vi "Begin.vi"(8 "error in":errorcluster) -> (0 "error out":errorcluster)   [LabVIEW 2017]
doc: "Called before other user functions, this VI is expected to open initial I/O refnums, load in file data, and do all program initialization. Notice that the <B>error out</B> terminal is simply used for data flow. Wiring it to other structures or subVIs ensures that this VI runs first."
uses:
  <vilib>/Rock Robotics/WPI/DriverStation/WPI_DriverStationRobotMode2.ctl
  TypeDef/CLUSTER_Arm_Device_IDs.ctl
  TypeDef/CLUSTER_Talon_Setup.ctl
  _SHARE ALL/RoboRio Share All/SRX Share All/TypeDefs SRX/Cluster_SRX_OPEN Data.ctl
  _SHARE ALL/RoboRio Share All/SRX Share All/TypeDefs SRX/Cluster_SRX_Current Config.ctl
  _SHARE ALL/RoboRio Share All/SRX Share All/TypeDefs SRX/Cluster_SRX_Sensor Config.ctl
  System Drivers/Phoenix-LabVIEW/Motor Controller/Controls/CTRE_Phoenix_MotorControl_FeedbackDevice.ctl
  _SHARE ALL/RoboRio Share All/SRX Share All/TypeDefs SRX/Cluster_SRX_Config Hard Limits.ctl
  System Drivers/Phoenix-LabVIEW/Motor Controller/Controls/CTRE_Phoenix_MotorControl_LimitSwitchNormal.ctl
  _SHARE ALL/RoboRio Share All/SRX Share All/TypeDefs SRX/Cluster_SRX_Motion Magic Config Data.ctl
  _SHARE ALL/RoboRio Share All/SRX Share All/TypeDefs SRX/Cluster_SRX_PIDF.ctl
  _SHARE ALL/RoboRio Share All/SRX Share All/TypeDefs SRX/Cluster_SRX_Config Soft Limits.ctl
  _SHARE ALL/RoboRio Share All/SRX Share All/TypeDefs SRX/Cluster_SRX_Config Voltage Output.ctl
  System Drivers/Phoenix-LabVIEW/Motor Controller/Controls/CTRE_Phoenix_MotorControl_NeutralMode.ctl
  _SHARE ALL/RoboRio Share All/SRX Share All/TypeDefs SRX/Cluster_SRX_Forward and Reverse.ctl
  TypeDef/CLUSTER_Claw_Setup.ctl
  TypeDef/CLUSTER_PWM Motor Setup.ctl
  <vilib>/Rock Robotics/SystemInterfaces/DIO/FPGA_DIOPWMChannel.ctl
  TypeDef/CLUSTER_Solonoid_Setup.ctl
  <vilib>/Rock Robotics/WPI/Solenoid/WPI_SolenoidChannel.ctl
  <vilib>/Rock Robotics/SystemInterfaces/DIO/FPGA_DIOChannel.ctl
  Robot Global Data.vi
  _SHARE ALL/Global Share All/Global_STOP.vi
  Globals/Global_Device_IDs.vi
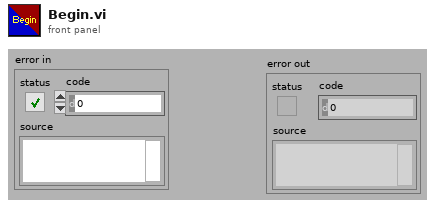
[diagram p1: front panel]
types:
  T1 = typedef "WPI_DriverStationRobotMode2.ctl" = enum16{"Autonomous Disabled", "Autonomous Enabled", "Teleop Disabled", "Teleop Enabled", "Disconnected", "Finish", "Test Disabled", "Test Enabled", "Emergency Stopped"}
  T2 = typedef "Cluster_SRX_Forward and Reverse.ctl" = cluster{"Forward":dbl, "Reverse":dbl}
  T3 = typedef "CTRE_Phoenix_MotorControl_NeutralMode.ctl" = enum8{"EEPROMSetting", "Override to Coast", "Override to Brake"}
  T4 = typedef "Cluster_SRX_Config Voltage Output.ctl" = cluster{"Invert?":bool, "Neutral Mode":T3, "Deadband (-1to1)":dbl, "Ramp Time Off to Full (S)":dbl, "Peak  (-1to1)":T2, "Nominal  (-1to1)":T2}
  T5 = typedef "Cluster_SRX_Config Soft Limits.ctl" = cluster{"Max":i32, "Min":i32, "Max Enable":bool, "Min Enable":bool}
  T6 = typedef "Cluster_SRX_PIDF.ctl" = cluster{"P":dbl, "I":dbl, "D":dbl, "F":dbl, "I Zone":dbl}
  T7 = typedef "Cluster_SRX_Sensor Config.ctl" = cluster{"Feedback Device":T8, "PhaseSensor":bool}
  T8 = typedef "CTRE_Phoenix_MotorControl_FeedbackDevice.ctl" = i8
  T9 = typedef "Cluster_SRX_OPEN Data.ctl" = cluster{"SRX ID":u8, "Invert Output":bool}
  T10 = typedef "CLUSTER_Talon_Setup.ctl" = cluster{"Open Data":T9, "Current Config Data":T11, "Sensor Config":T7, "Hard Limits":T12, "Motion Magic Config Data":T14, "PIDF":T6, "Maximum Integral Accumulator Value":dbl, "AllowableClosedLoop":i32, "Limits":T5, "Output Config":T4}
  T11 = typedef "Cluster_SRX_Current Config.ctl" = cluster{"Enable Current Limit?":bool, "Peak Current (Amps)":i32, "Peak Current Maximum Duration (ms)":i32, "Continuous Current Limit (Amps)":i32}
  T12 = typedef "Cluster_SRX_Config Hard Limits.ctl" = cluster{"Fwd Enable":bool, "Rev Enable":bool, "Fwd NO-NC":T13, "Rev NO-NC":T13}
  T13 = typedef "CTRE_Phoenix_MotorControl_LimitSwitchNormal.ctl" = enum16{"Normally Open", "Normally Closed", "Disabled"}
  T14 = typedef "Cluster_SRX_Motion Magic Config Data.ctl" = cluster{"Cruise Velocity":i32, "Acceleration":i32}
  T15 = typedef "CLUSTER_Arm_Device_IDs.ctl" = cluster{"Master":T10, "Slave":T10}
  T16 = typedef "FPGA_DIOChannel.ctl" = enum8{"DIO 0", "DIO 1", "DIO 2", "DIO 3", "DIO 4", "DIO 5", "DIO 6", "DIO 7", "DIO 8", "DIO 9", "DIO MXP 0", "DIO MXP 1", "DIO MXP 2", "DIO MXP 3", "DIO MXP 4", "DIO MXP 5", "DIO MXP 6", "DIO MXP 7", "DIO MXP 8", "DIO MXP 9", "DIO MXP 10", "DIO MXP 11", "DIO MXP 12", "DIO MXP 13", "DIO MXP 14", "DIO MXP 15", "SPI Port CS1", "SPI Port CS2", "SPI Port CS3", "SPI Port MISO", "SPI Port MOSI", "Invalid"}
  T17 = typedef "WPI_SolenoidChannel.ctl" = enum8{"Solenoid 0", "Solenoid 1", "Solenoid 2", "Solenoid 3", "Solenoid 4", "Solenoid 5", "Solenoid 6", "Solenoid 7", "Invalid"}
  T18 = typedef "FPGA_DIOPWMChannel.ctl" = enum8{"PWM 0", "PWM 1", "PWM 2", "PWM 3", "PWM 4", "PWM 5", "PWM 6", "PWM 7", "PWM 8", "PWM 9", "PWM MXP 0", "PWM MXP 1", "PWM MXP 2", "PWM MXP 3", "PWM MXP 4", "PWM MXP 5", "PWM MXP 6", "PWM MXP 7", "PWM MXP 8", "PWM MXP 9", "Invalid"}
  T19 = typedef "CLUSTER_Claw_Setup.ctl" = cluster{"Left Motor Setup":T20, "Right Motor Setup":T20, "Left Motor PDP":i32, "Right Motor PDP":i32, "Solonoid Setup":T21, "Limit Switch DIO":T16}
  T20 = typedef "CLUSTER_PWM Motor Setup.ctl" = cluster{"Motor PWM":T18, "Invert Motor":bool}
  T21 = typedef "CLUSTER_Solonoid_Setup.ctl" = cluster{"Pneumatics Control Module (0)":u8, "Forward Solenoid Channel":T17, "Reverse Solenoid Channel":T17}
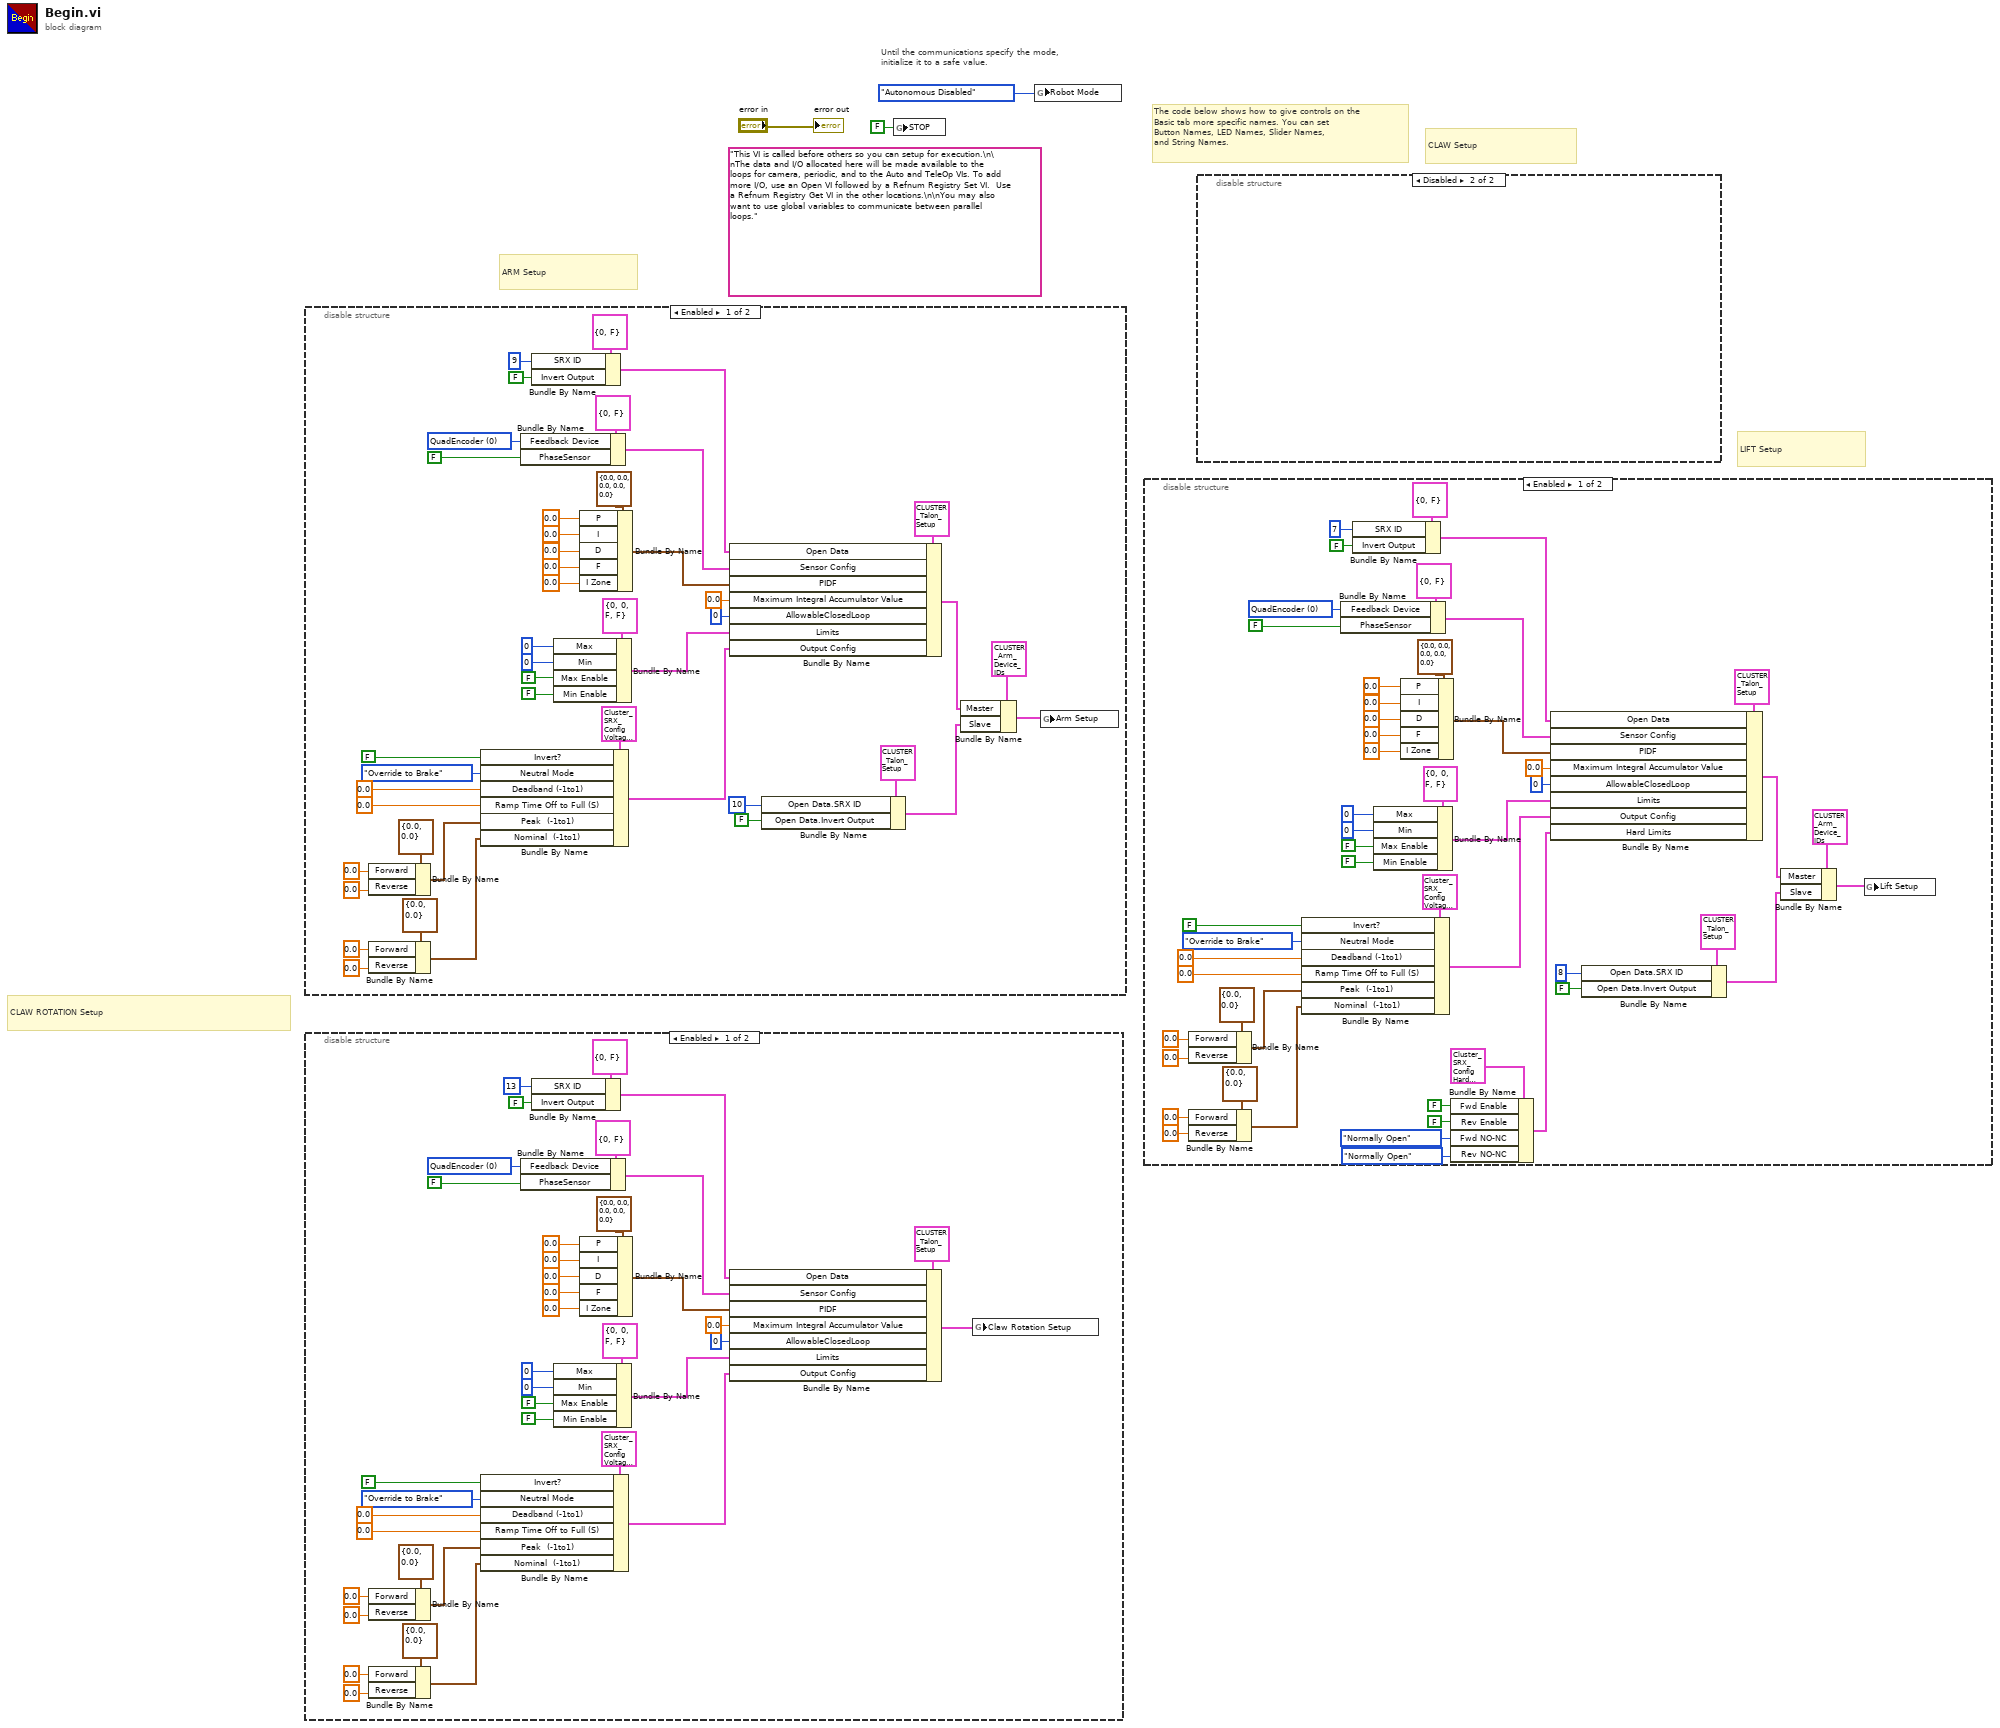
[diagram p0: block diagram]
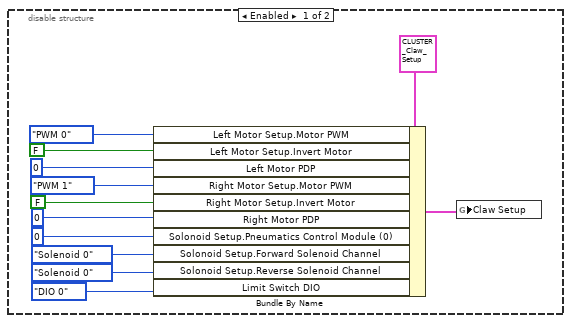
[diagram p4: hidden frame]
diagram:
  (unwired) "This VI is called before others so you can setup for execution.\n\nThe data and I/O allocated here will be made available to the loops for camera, periodic, and to the Auto and TeleOp VIs. To add more I/O, use an Open VI followed by a Refnum Registry Set VI.  Use a Refnum Registry Get VI in the other locations.\n\nYou may also want to use global variables to communicate between parallel loops."
  # "CLAW ROTATION Setup"
  # "LIFT Setup"
  # "CLAW Setup"
  # "ARM Setup"
  # "The code below shows how to give controls on the\nBasic tab more specific names. You can set\nButton Names, LED Names, Slider Names,\nand String Names."
  # "Until the communications specify the mode,\ninitialize it to a safe value."
  n1 = disable-structure shown="Enabled" {
    frame Enabled {
      w28 = T8 0 items=["None"=-1, "QuadEncoder"=0, "Analog"=2, "Tachometer"=4, "Pulse Width Encoded Position"=8, "Sensor Sum (S0 + S1)"=9, "Sensor Difference (D0 - D1)"=10, "Remote Source 0"=11, "Remote Source 1"=12, "Software Emulated"=15] ("Feedback Device")
      n2 = Bundle By Name(cluster=T2 {"Forward"=0.0, "Reverse"=0.0} ("Peak  (-1to1)"), "Forward"=0.0, "Reverse"=0.0) -> (w12:T2)
      n3 = Bundle By Name(cluster=T2 {"Forward"=0.0, "Reverse"=0.0} ("Nominal  (-1to1)"), "Forward"=0.0, "Reverse"=0.0) -> (w10:T2)
      n4 = Bundle By Name(cluster=T4 {"Invert?"=FALSE, "Neutral Mode"=enum."Override to Coast", "Deadband (-1to1)"=0.0, "Ramp Time Off to Full (S)"=0.0, "Peak  (-1to1)"={"Forward"=1.0, "Reverse"=-1.0}, "Nominal  (-1to1)"={"Forward"=0.0, "Reverse"=0.0}} ("Output Config"), "Invert?"=FALSE, "Neutral Mode"=CTRE_Phoenix_MotorControl_NeutralMode."Override to Brake", "Deadband (-1to1)"=0.0, "Ramp Time Off to Full (S)"=0.0, "Peak  (-1to1)"=w12, "Nominal  (-1to1)"=w10) -> (w31:T4)
      n5 = Bundle By Name(cluster=T7 {"Feedback Device"=0, "PhaseSensor"=FALSE} ("Sensor Config"), "Feedback Device"=w28, "PhaseSensor"=FALSE) -> (w39:T7)
      n6 = Bundle By Name(cluster=T9 {"SRX ID"=0, "Invert Output"=FALSE} ("Open Data"), "SRX ID"=u8 9, "Invert Output"=FALSE) -> (w41:T9)
      n7 = Bundle By Name(cluster=T5 {"Max"=0, "Min"=0, "Max Enable"=FALSE, "Min Enable"=FALSE} ("Limits"), "Max"=0, "Min"=0, "Max Enable"=FALSE, "Min Enable"=FALSE) -> (w33:T5)
      n8 = Bundle By Name(cluster=T6 {"P"=0.0, "I"=0.0, "D"=0.0, "F"=0.0, "I Zone"=0.0} ("PIDF"), "P"=0.0, "I"=0.0, "D"=0.0, "F"=0.0, "I Zone"=0.0) -> (w37:T6)
      n9 = Bundle By Name(cluster=T10 {"Open Data"={"SRX ID"=0, "Invert Output"=FALSE}, "Current Config Data"={"Enable Current Limit?"=FALSE, "Peak Current (Amps)"=0, "Peak Current Maximum Duration (ms)"=0, "Continuous Current Limit (Amps)"=0}, "Sensor Config"={"Feedback Device"=0, "PhaseSensor"=FALSE}, "Hard Limits"={"Fwd Enable"=FALSE, "Rev Enable"=FALSE, "Fwd NO-NC"=enum."Normally Open", "Rev NO-NC"=enum."Normally Open"}, "Motion Magic Config Data"={"Cruise Velocity"=0, "Acceleration"=0}, "PIDF"={"P"=0.0, "I"=0.0, "D"=0.0, "F"=0.0, "I Zone"=0.0}, "Maximum Integral Accumulator Value"=0.0, "AllowableClosedLoop"=0, "Limits"={"Max"=0, "Min"=0, "Max Enable"=FALSE, "Min Enable"=FALSE}, "Output Config"={"Invert?"=FALSE, "Neutral Mode"=enum."Override to Coast", "Deadband (-1to1)"=0.0, "Ramp Time Off to Full (S)"=0.0, "Peak  (-1to1)"={"Forward"=1.0, "Reverse"=-1.0}, "Nominal  (-1to1)"={"Forward"=0.0, "Reverse"=0.0}}} ("Master"), "Open Data"=w41, "Sensor Config"=w39, "PIDF"=w37, "Maximum Integral Accumulator Value"=0.0, "AllowableClosedLoop"=0, "Limits"=w33, "Output Config"=w31) -> (w45:T10)
      n10 = Bundle By Name(cluster=T10 {"Open Data"={"SRX ID"=0, "Invert Output"=FALSE}, "Current Config Data"={"Enable Current Limit?"=FALSE, "Peak Current (Amps)"=0, "Peak Current Maximum Duration (ms)"=0, "Continuous Current Limit (Amps)"=0}, "Sensor Config"={"Feedback Device"=0, "PhaseSensor"=FALSE}, "Hard Limits"={"Fwd Enable"=FALSE, "Rev Enable"=FALSE, "Fwd NO-NC"=enum."Normally Open", "Rev NO-NC"=enum."Normally Open"}, "Motion Magic Config Data"={"Cruise Velocity"=0, "Acceleration"=0}, "PIDF"={"P"=0.0, "I"=0.0, "D"=0.0, "F"=0.0, "I Zone"=0.0}, "Maximum Integral Accumulator Value"=0.0, "AllowableClosedLoop"=0, "Limits"={"Max"=0, "Min"=0, "Max Enable"=FALSE, "Min Enable"=FALSE}, "Output Config"={"Invert?"=FALSE, "Neutral Mode"=enum."Override to Coast", "Deadband (-1to1)"=0.0, "Ramp Time Off to Full (S)"=0.0, "Peak  (-1to1)"={"Forward"=1.0, "Reverse"=-1.0}, "Nominal  (-1to1)"={"Forward"=0.0, "Reverse"=0.0}}} ("Master"), "Open Data.SRX ID"=u8 10, "Open Data.Invert Output"=FALSE) -> (w44:T10)
      n11 = Bundle By Name(cluster=T15 {"Master"={"Open Data"={"SRX ID"=0, "Invert Output"=FALSE}, "Current Config Data"={"Enable Current Limit?"=FALSE, "Peak Current (Amps)"=0, "Peak Current Maximum Duration (ms)"=2, "Continuous Current Limit (Amps)"=0}, "Sensor Config"={"Feedback Device"=0, "PhaseSensor"=FALSE}, "Hard Limits"={"Fwd Enable"=FALSE, "Rev Enable"=FALSE, "Fwd NO-NC"=enum."Normally Open", "Rev NO-NC"=enum."Normally Open"}, "Motion Magic Config Data"={"Cruise Velocity"=0, "Acceleration"=0}, "PIDF"={"P"=0.0, "I"=0.0, "D"=0.0, "F"=0.0, "I Zone"=0.0}, "Maximum Integral Accumulator Value"=0.0, "AllowableClosedLoop"=0, "Limits"={"Max"=0, "Min"=0, "Max Enable"=FALSE, "Min Enable"=FALSE}, "Output Config"={"Invert?"=FALSE, "Neutral Mode"=enum."Override to Coast", "Deadband (-1to1)"=0.0, "Ramp Time Off to Full (S)"=0.0, "Peak  (-1to1)"={"Forward"=1.0, "Reverse"=-1.0}, "Nominal  (-1to1)"={"Forward"=0.0, "Reverse"=0.0}}}, "Slave"={"Open Data"={"SRX ID"=0, "Invert Output"=FALSE}, "Current Config Data"={"Enable Current Limit?"=FALSE, "Peak Current (Amps)"=0, "Peak Current Maximum Duration (ms)"=-1, "Continuous Current Limit (Amps)"=0}, "Sensor Config"={"Feedback Device"=0, "PhaseSensor"=FALSE}, "Hard Limits"={"Fwd Enable"=FALSE, "Rev Enable"=FALSE, "Fwd NO-NC"=enum."Normally Open", "Rev NO-NC"=enum."Normally Open"}, "Motion Magic Config Data"={"Cruise Velocity"=0, "Acceleration"=0}, "PIDF"={"P"=0.0, "I"=0.0, "D"=0.0, "F"=0.0, "I Zone"=0.0}, "Maximum Integral Accumulator Value"=0.0, "AllowableClosedLoop"=0, "Limits"={"Max"=0, "Min"=0, "Max Enable"=FALSE, "Min Enable"=FALSE}, "Output Config"={"Invert?"=FALSE, "Neutral Mode"=enum."Override to Coast", "Deadband (-1to1)"=0.0, "Ramp Time Off to Full (S)"=0.0, "Peak  (-1to1)"={"Forward"=1.0, "Reverse"=-1.0}, "Nominal  (-1to1)"={"Forward"=0.0, "Reverse"=0.0}}}} ("Arm Setup"), "Master"=w45, "Slave"=w44) -> (w47:T15)
      n12 = global write "Global_Device_IDs.vi" "Arm Setup"(w47) -> ()
    }
    frame Disabled {
    }
  }
  n13 = disable-structure shown="Enabled" {
    frame Enabled {
      w72 = T8 0 items=["None"=-1, "QuadEncoder"=0, "Analog"=2, "Tachometer"=4, "Pulse Width Encoded Position"=8, "Sensor Sum (S0 + S1)"=9, "Sensor Difference (D0 - D1)"=10, "Remote Source 0"=11, "Remote Source 1"=12, "Software Emulated"=15] ("Feedback Device")
      n14 = Bundle By Name(cluster=T2 {"Forward"=0.0, "Reverse"=0.0} ("Peak  (-1to1)"), "Forward"=0.0, "Reverse"=0.0) -> (w56:T2)
      n15 = Bundle By Name(cluster=T2 {"Forward"=0.0, "Reverse"=0.0} ("Nominal  (-1to1)"), "Forward"=0.0, "Reverse"=0.0) -> (w54:T2)
      n16 = Bundle By Name(cluster=T4 {"Invert?"=FALSE, "Neutral Mode"=enum."Override to Coast", "Deadband (-1to1)"=0.0, "Ramp Time Off to Full (S)"=0.0, "Peak  (-1to1)"={"Forward"=1.0, "Reverse"=-1.0}, "Nominal  (-1to1)"={"Forward"=0.0, "Reverse"=0.0}} ("Output Config"), "Invert?"=FALSE, "Neutral Mode"=CTRE_Phoenix_MotorControl_NeutralMode."Override to Brake", "Deadband (-1to1)"=0.0, "Ramp Time Off to Full (S)"=0.0, "Peak  (-1to1)"=w56, "Nominal  (-1to1)"=w54) -> (w75:T4)
      n17 = Bundle By Name(cluster=T7 {"Feedback Device"=0, "PhaseSensor"=FALSE} ("Sensor Config"), "Feedback Device"=w72, "PhaseSensor"=FALSE) -> (w83:T7)
      n18 = Bundle By Name(cluster=T9 {"SRX ID"=0, "Invert Output"=FALSE} ("Open Data"), "SRX ID"=u8 13, "Invert Output"=FALSE) -> (w85:T9)
      n19 = Bundle By Name(cluster=T5 {"Max"=0, "Min"=0, "Max Enable"=FALSE, "Min Enable"=FALSE} ("Limits"), "Max"=0, "Min"=0, "Max Enable"=FALSE, "Min Enable"=FALSE) -> (w77:T5)
      n20 = Bundle By Name(cluster=T6 {"P"=0.0, "I"=0.0, "D"=0.0, "F"=0.0, "I Zone"=0.0} ("PIDF"), "P"=0.0, "I"=0.0, "D"=0.0, "F"=0.0, "I Zone"=0.0) -> (w81:T6)
      n21 = Bundle By Name(cluster=T10 {"Open Data"={"SRX ID"=0, "Invert Output"=FALSE}, "Current Config Data"={"Enable Current Limit?"=FALSE, "Peak Current (Amps)"=0, "Peak Current Maximum Duration (ms)"=0, "Continuous Current Limit (Amps)"=0}, "Sensor Config"={"Feedback Device"=0, "PhaseSensor"=FALSE}, "Hard Limits"={"Fwd Enable"=FALSE, "Rev Enable"=FALSE, "Fwd NO-NC"=enum."Normally Open", "Rev NO-NC"=enum."Normally Open"}, "Motion Magic Config Data"={"Cruise Velocity"=0, "Acceleration"=0}, "PIDF"={"P"=0.0, "I"=0.0, "D"=0.0, "F"=0.0, "I Zone"=0.0}, "Maximum Integral Accumulator Value"=0.0, "AllowableClosedLoop"=0, "Limits"={"Max"=0, "Min"=0, "Max Enable"=FALSE, "Min Enable"=FALSE}, "Output Config"={"Invert?"=FALSE, "Neutral Mode"=enum."Override to Coast", "Deadband (-1to1)"=0.0, "Ramp Time Off to Full (S)"=0.0, "Peak  (-1to1)"={"Forward"=1.0, "Reverse"=-1.0}, "Nominal  (-1to1)"={"Forward"=0.0, "Reverse"=0.0}}} ("Master"), "Open Data"=w85, "Sensor Config"=w83, "PIDF"=w81, "Maximum Integral Accumulator Value"=0.0, "AllowableClosedLoop"=0, "Limits"=w77, "Output Config"=w75) -> (w49:T10)
      n22 = global write "Global_Device_IDs.vi" "Claw Rotation Setup"(w49) -> ()
    }
    frame Disabled {
    }
  }
  n23 = global write "Global_STOP.vi" "STOP"(FALSE ("STOP")) -> ()
  n24 = global write "Robot Global Data.vi" "Robot Mode"(WPI_DriverStationRobotMode2."Autonomous Disabled" ("Robot Mode")) -> ()
  n25 = disable-structure shown="Enabled" {
    frame Enabled {
      w118 = T8 0 items=["None"=-1, "QuadEncoder"=0, "Analog"=2, "Tachometer"=4, "Pulse Width Encoded Position"=8, "Sensor Sum (S0 + S1)"=9, "Sensor Difference (D0 - D1)"=10, "Remote Source 0"=11, "Remote Source 1"=12, "Software Emulated"=15] ("Feedback Device")
      n26 = Bundle By Name(cluster=T2 {"Forward"=0.0, "Reverse"=0.0} ("Peak  (-1to1)"), "Forward"=0.0, "Reverse"=0.0) -> (w102:T2)
      n27 = Bundle By Name(cluster=T2 {"Forward"=0.0, "Reverse"=0.0} ("Nominal  (-1to1)"), "Forward"=0.0, "Reverse"=0.0) -> (w100:T2)
      n28 = Bundle By Name(cluster=T4 {"Invert?"=FALSE, "Neutral Mode"=enum."Override to Coast", "Deadband (-1to1)"=0.0, "Ramp Time Off to Full (S)"=0.0, "Peak  (-1to1)"={"Forward"=1.0, "Reverse"=-1.0}, "Nominal  (-1to1)"={"Forward"=0.0, "Reverse"=0.0}} ("Output Config"), "Invert?"=FALSE, "Neutral Mode"=CTRE_Phoenix_MotorControl_NeutralMode."Override to Brake", "Deadband (-1to1)"=0.0, "Ramp Time Off to Full (S)"=0.0, "Peak  (-1to1)"=w102, "Nominal  (-1to1)"=w100) -> (w121:T4)
      n29 = Bundle By Name(cluster=T7 {"Feedback Device"=0, "PhaseSensor"=FALSE} ("Sensor Config"), "Feedback Device"=w118, "PhaseSensor"=FALSE) -> (w129:T7)
      n30 = Bundle By Name(cluster=T9 {"SRX ID"=0, "Invert Output"=FALSE} ("Open Data"), "SRX ID"=u8 7, "Invert Output"=FALSE) -> (w131:T9)
      n31 = Bundle By Name(cluster=T5 {"Max"=0, "Min"=0, "Max Enable"=FALSE, "Min Enable"=FALSE} ("Limits"), "Max"=0, "Min"=0, "Max Enable"=FALSE, "Min Enable"=FALSE) -> (w123:T5)
      n32 = Bundle By Name(cluster=T6 {"P"=0.0, "I"=0.0, "D"=0.0, "F"=0.0, "I Zone"=0.0} ("PIDF"), "P"=0.0, "I"=0.0, "D"=0.0, "F"=0.0, "I Zone"=0.0) -> (w127:T6)
      n33 = Bundle By Name(cluster=T12 {"Fwd Enable"=FALSE, "Rev Enable"=FALSE, "Fwd NO-NC"=enum."Normally Open", "Rev NO-NC"=enum."Normally Open"} ("Hard Limits"), "Fwd Enable"=FALSE, "Rev Enable"=FALSE, "Fwd NO-NC"=CTRE_Phoenix_MotorControl_LimitSwitchNormal."Normally Open", "Rev NO-NC"=CTRE_Phoenix_MotorControl_LimitSwitchNormal."Normally Open") -> (w93:T12)
      n34 = Bundle By Name(cluster=T10 {"Open Data"={"SRX ID"=0, "Invert Output"=FALSE}, "Current Config Data"={"Enable Current Limit?"=FALSE, "Peak Current (Amps)"=0, "Peak Current Maximum Duration (ms)"=0, "Continuous Current Limit (Amps)"=0}, "Sensor Config"={"Feedback Device"=0, "PhaseSensor"=FALSE}, "Hard Limits"={"Fwd Enable"=FALSE, "Rev Enable"=FALSE, "Fwd NO-NC"=enum."Normally Open", "Rev NO-NC"=enum."Normally Open"}, "Motion Magic Config Data"={"Cruise Velocity"=0, "Acceleration"=0}, "PIDF"={"P"=0.0, "I"=0.0, "D"=0.0, "F"=0.0, "I Zone"=0.0}, "Maximum Integral Accumulator Value"=0.0, "AllowableClosedLoop"=0, "Limits"={"Max"=0, "Min"=0, "Max Enable"=FALSE, "Min Enable"=FALSE}, "Output Config"={"Invert?"=FALSE, "Neutral Mode"=enum."Override to Coast", "Deadband (-1to1)"=0.0, "Ramp Time Off to Full (S)"=0.0, "Peak  (-1to1)"={"Forward"=1.0, "Reverse"=-1.0}, "Nominal  (-1to1)"={"Forward"=0.0, "Reverse"=0.0}}} ("Master"), "Open Data"=w131, "Sensor Config"=w129, "PIDF"=w127, "Maximum Integral Accumulator Value"=0.0, "AllowableClosedLoop"=0, "Limits"=w123, "Output Config"=w121, "Hard Limits"=w93) -> (w135:T10)
      n35 = Bundle By Name(cluster=T10 {"Open Data"={"SRX ID"=0, "Invert Output"=FALSE}, "Current Config Data"={"Enable Current Limit?"=FALSE, "Peak Current (Amps)"=0, "Peak Current Maximum Duration (ms)"=0, "Continuous Current Limit (Amps)"=0}, "Sensor Config"={"Feedback Device"=0, "PhaseSensor"=FALSE}, "Hard Limits"={"Fwd Enable"=FALSE, "Rev Enable"=FALSE, "Fwd NO-NC"=enum."Normally Open", "Rev NO-NC"=enum."Normally Open"}, "Motion Magic Config Data"={"Cruise Velocity"=0, "Acceleration"=0}, "PIDF"={"P"=0.0, "I"=0.0, "D"=0.0, "F"=0.0, "I Zone"=0.0}, "Maximum Integral Accumulator Value"=0.0, "AllowableClosedLoop"=0, "Limits"={"Max"=0, "Min"=0, "Max Enable"=FALSE, "Min Enable"=FALSE}, "Output Config"={"Invert?"=FALSE, "Neutral Mode"=enum."Override to Coast", "Deadband (-1to1)"=0.0, "Ramp Time Off to Full (S)"=0.0, "Peak  (-1to1)"={"Forward"=1.0, "Reverse"=-1.0}, "Nominal  (-1to1)"={"Forward"=0.0, "Reverse"=0.0}}} ("Master"), "Open Data.SRX ID"=u8 8, "Open Data.Invert Output"=FALSE) -> (w134:T10)
      n36 = Bundle By Name(cluster=T15 {"Master"={"Open Data"={"SRX ID"=0, "Invert Output"=FALSE}, "Current Config Data"={"Enable Current Limit?"=FALSE, "Peak Current (Amps)"=0, "Peak Current Maximum Duration (ms)"=2, "Continuous Current Limit (Amps)"=0}, "Sensor Config"={"Feedback Device"=0, "PhaseSensor"=FALSE}, "Hard Limits"={"Fwd Enable"=FALSE, "Rev Enable"=FALSE, "Fwd NO-NC"=enum."Normally Open", "Rev NO-NC"=enum."Normally Open"}, "Motion Magic Config Data"={"Cruise Velocity"=0, "Acceleration"=0}, "PIDF"={"P"=0.0, "I"=0.0, "D"=0.0, "F"=0.0, "I Zone"=0.0}, "Maximum Integral Accumulator Value"=0.0, "AllowableClosedLoop"=0, "Limits"={"Max"=0, "Min"=0, "Max Enable"=FALSE, "Min Enable"=FALSE}, "Output Config"={"Invert?"=FALSE, "Neutral Mode"=enum."Override to Coast", "Deadband (-1to1)"=0.0, "Ramp Time Off to Full (S)"=0.0, "Peak  (-1to1)"={"Forward"=1.0, "Reverse"=-1.0}, "Nominal  (-1to1)"={"Forward"=0.0, "Reverse"=0.0}}}, "Slave"={"Open Data"={"SRX ID"=0, "Invert Output"=FALSE}, "Current Config Data"={"Enable Current Limit?"=FALSE, "Peak Current (Amps)"=0, "Peak Current Maximum Duration (ms)"=-1, "Continuous Current Limit (Amps)"=0}, "Sensor Config"={"Feedback Device"=0, "PhaseSensor"=FALSE}, "Hard Limits"={"Fwd Enable"=FALSE, "Rev Enable"=FALSE, "Fwd NO-NC"=enum."Normally Open", "Rev NO-NC"=enum."Normally Open"}, "Motion Magic Config Data"={"Cruise Velocity"=0, "Acceleration"=0}, "PIDF"={"P"=0.0, "I"=0.0, "D"=0.0, "F"=0.0, "I Zone"=0.0}, "Maximum Integral Accumulator Value"=0.0, "AllowableClosedLoop"=0, "Limits"={"Max"=0, "Min"=0, "Max Enable"=FALSE, "Min Enable"=FALSE}, "Output Config"={"Invert?"=FALSE, "Neutral Mode"=enum."Override to Coast", "Deadband (-1to1)"=0.0, "Ramp Time Off to Full (S)"=0.0, "Peak  (-1to1)"={"Forward"=1.0, "Reverse"=-1.0}, "Nominal  (-1to1)"={"Forward"=0.0, "Reverse"=0.0}}}} ("Arm Setup"), "Master"=w135, "Slave"=w134) -> (w137:T15)
      n37 = global write "Global_Device_IDs.vi" "Lift Setup"(w137) -> ()
    }
    frame Disabled {
    }
  }
  n38 = disable-structure shown="Disabled" {
    frame Enabled {
      n39 = Bundle By Name(cluster=T19 {"Left Motor Setup"={"Motor PWM"=enum."PWM 0", "Invert Motor"=FALSE}, "Right Motor Setup"={"Motor PWM"=enum."PWM 0", "Invert Motor"=FALSE}, "Left Motor PDP"=0, "Right Motor PDP"=0, "Solonoid Setup"={"Pneumatics Control Module (0)"=0, "Forward Solenoid Channel"=enum."Solenoid 0", "Reverse Solenoid Channel"=enum."Solenoid 0"}, "Limit Switch DIO"=enum."DIO 0"} ("Claw Setup"), "Left Motor Setup.Motor PWM"=FPGA_DIOPWMChannel."PWM 0", "Left Motor Setup.Invert Motor"=FALSE, "Left Motor PDP"=0, "Right Motor Setup.Motor PWM"=FPGA_DIOPWMChannel."PWM 1", "Right Motor Setup.Invert Motor"=FALSE, "Right Motor PDP"=0, "Solonoid Setup.Pneumatics Control Module (0)"=u8 0, "Solonoid Setup.Forward Solenoid Channel"=WPI_SolenoidChannel."Solenoid 0", "Solonoid Setup.Reverse Solenoid Channel"=WPI_SolenoidChannel."Solenoid 0", "Limit Switch DIO"=FPGA_DIOChannel."DIO 0") -> (w149:T19)
      n40 = global write "Global_Device_IDs.vi" "Claw Setup"(w149) -> ()
    }
    frame Disabled {
    }
  }
  "error out" <- "error in"
